vi "Enumerate video codecs.vi"(3 "Codec Source":T1 items=["Default", "System", "Built in Vision"]) -> (0 "Error Out":errorcluster, 1 "Codec Names":string[](array[string]))   [LabVIEW 2014]
uses:
  <vilib>/vision/Avi.llb/IMAQ AVI2 Codec Path.ctl
panel:
  # "PN 27/11/2014"
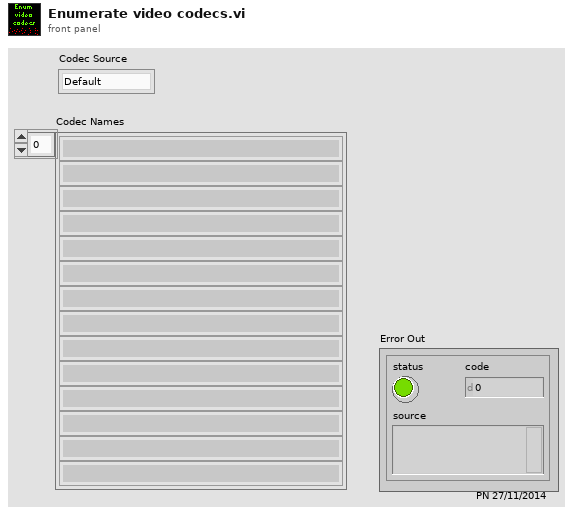
[diagram p1: front panel]
types:
  T1 = typedef "IMAQ AVI2 Codec Path.ctl" = u32
  T2 = typedef "Image Type" = u32
  T3 = typedef "IMAQ Image.ctl" = refnum<image>
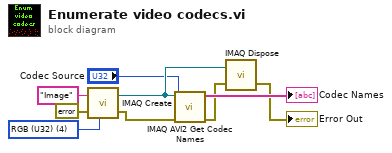
[diagram p0: block diagram]
diagram:
  w8 = T2 4 items=["Grayscale (U8)", "Grayscale (I16)", "Grayscale (SGL)", "Complex (CSG)", "RGB (U32)", "HSL (U32)", "RGB (U64)", "Grayscale (U16)"] ("Image Type")
  n1 = call "IMAQ Create"("Image Name"="Image", "Image Type"=w8, "error in (no error)"=errorcluster {"status"=FALSE, "code"=0, "source"=""} ("error in")) -> ("New Image"=w5:T3, "error out"=w7:errorcluster)  [unwired: 2 in]
  n2 = call "IMAQ AVI2 Get Codec Names"("error in (no error)"=w7, "Codec Source"="Codec Source", "Image"=w5) -> ("error out"=w4:errorcluster, "Codec Names"=→"Codec Names":string[])  [unwired: 7 in]
  n3 = call "IMAQ Dispose"("Image"=w5, "error in (no error)"=w4) -> ("error out"=→"Error Out":errorcluster)  [unwired: 4 in]
